vi "LEBITplc.TestIonSourceMonitor.vi"(0 "i ref in":refnum<vi>, 1 "data":i8[](array[numeric]), 2 "i attribute in":T1, 3 "index":i32, 4 "NickNames":string, 5 "error in":errorcluster, 7 "no link":bool) -> (14 "i ref out":refnum<vi>, 15 "Data":dbl[](array[numeric]), 16 "i attribute out":T1, 17 "Indexs":i32[](array[numeric]), 19 "error out":errorcluster)   [LabVIEW 2014, in "LEBITplc.lvlib"]
uses:
  LEBITplc.lvlib
  LEBITplc.i attribute.ctl
panel:
  out "No Link":bool
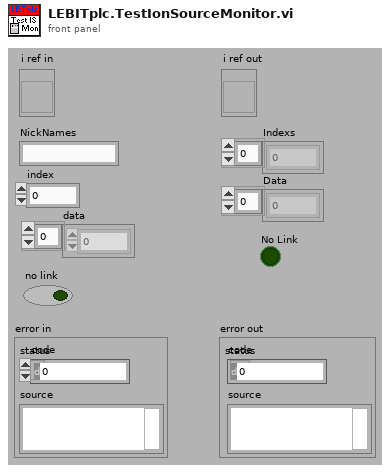
[diagram p1: front panel]
types:
  T1 = typedef "LEBITplc.lvlib/LEBITplc.i attribute.ctl" = cluster{"LLFLocation":string, "SetFileLocation":string, "nickNames":string[], "setValuePLCServiceID":i32[], "GUIServiceID":i32[], "monValuePLC":string[], "SetValueServiceID":i32[], "MonValueServiceID":i32[], "SetValue":dbl[][], "SetValueMin":dbl[], "SetValueMax":dbl[], "SetValueInfoServiceID":i32[], "GUINames":string[], "ListOfBases":string[], "Scale":dbl[], "Offset":dbl[], "setValuePLC":string[], "BaseName":string[], "ScaleServiceID":i32[], "OffsetServiceID":i32[], "AllPLCValues":string[], "CondSpecialArray":string[][], "CondSpecialIndex":i32[], "CondSpecialMonValue":dbl[], "RecentlyChanged":i32[], "SetFileLocationID":i32, "Dependent-Monitors":string[][], "LastLoadedFiles":string[], "IonGuideCalibLocation":string, "Monitor Dependent":string[], "Special":string[], "PLC?":bool[], "Start Date":string, "ListOfBasesServiceID":i32, "SETRA VISA resource":refnum<visa-resource-name>}
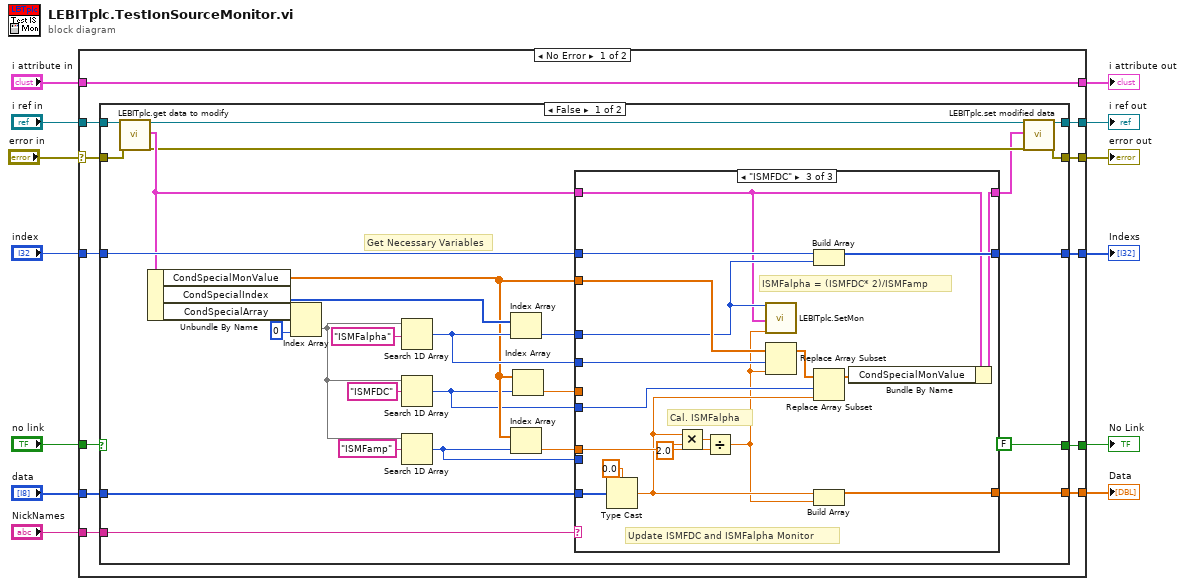
[diagram p0: block diagram]
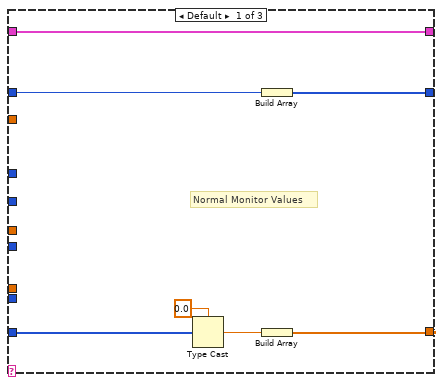
[diagram p2: hidden frame]
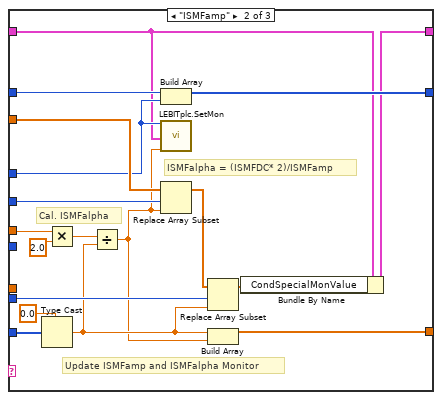
[diagram p3: hidden frame]
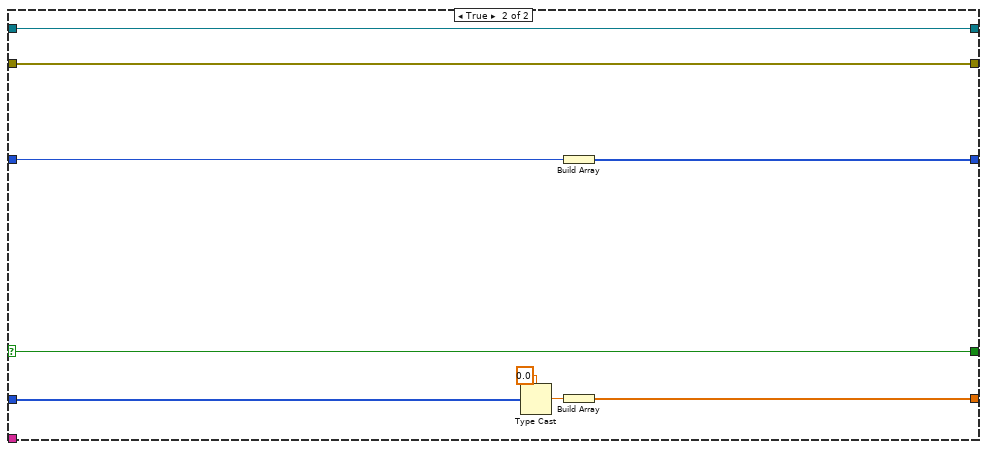
[diagram p4: hidden frame]
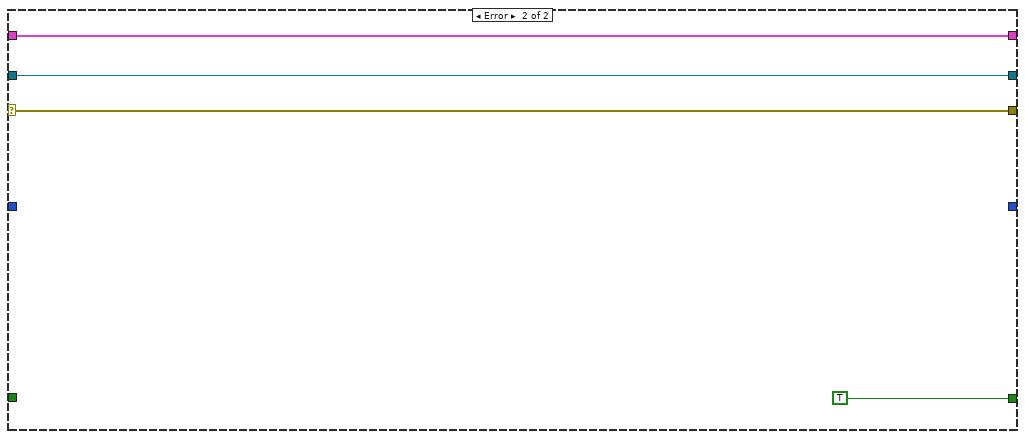
[diagram p5: hidden frame]
diagram:
  n1 = case shown="No Error" "error in" {
    selector: "error in" -> [w19 w109]
    tunnel: "NickNames" -> [w25 _]
    tunnel: [w20 w109] -> w12
    tunnel: "data" -> [w24 _]
    tunnel: "i attribute in" -> [w16 w107]
    tunnel: "i ref in" -> [w21 w108]
    tunnel: [w15 w108] -> w7
    tunnel: "index" -> [w23 _]
    tunnel: [w16 w107] -> w5
    tunnel: [w22 _] -> w4
    tunnel: "no link" -> [w18 _]
    tunnel: [w17 TRUE] -> w2
    tunnel: [w14 _] -> w1
    frame No Error {
      n2 = case shown="False" w18 {
        selector: w18 -> [_ w103]
        tunnel: w25 -> [w50 _]
        tunnel: w24 -> [w49 w99]
        tunnel: w23 -> [w42 w102]
        tunnel: [w41 w101] -> w22
        tunnel: w21 -> [w34 w105]
        tunnel: [w28 w105] -> w15
        tunnel: [w29 w104] -> w20
        tunnel: w19 -> [w32 w104]
        tunnel: [FALSE w103] -> w17
        tunnel: [w26 w97] -> w14
        frame False {
          # "Get Necessary Variables"
          n3 = call "LEBITplc.get data to modify.vi"("i ref in"=w34, "error in (no error)"=w32) -> ("i ref out"=w31:refnum<vi>, "i attribute"=w33:T1, "error out"=w30:errorcluster)  [unwired: 14 in, 1 out]
          n4 = Unbundle By Name(w33) -> ("CondSpecialMonValue"=w38:dbl[], "CondSpecialIndex"=w45:i32[], "CondSpecialArray"=w53:string[][])
          n5 = Index Array(array=w53, index (col)=0 ("index (row)")) -> (element=w44:string[])  [unwired: 1 in]
          n6 = Search 1D Array(1D array=w44, element="ISMFalpha") -> (index of element=w39:i32)  [unwired: 1 in]
          n7 = Search 1D Array(1D array=w44, element="ISMFDC") -> (index of element=w36:i32)  [unwired: 1 in]
          n8 = Search 1D Array(1D array=w44, element="ISMFamp") -> (index of element=w37:i32)  [unwired: 1 in]
          n9 = Index Array(array=w45, index=w39) -> (element=w43:i32)
          n10 = Index Array(array=w38, index=w37) -> (element=w46:dbl)
          n11 = Index Array(array=w38, index=w36) -> (element=w47:dbl)
          n12 = case shown="\"ISMFDC\"" w50 {
            tunnel: w49 -> [w57 w76 w94]
            tunnel: w47 -> [_ w68 _]
            tunnel: w46 -> [_ _ w85]
            tunnel: w43 -> [_ w62 w81]
            tunnel: w42 -> [w59 w77 w95]
            tunnel: [w60 w75 w93] -> w41
            tunnel: w33 -> [w54 w61 w80]
            tunnel: [w54 w70 w89] -> w27
            tunnel: w39 -> [_ w74 w92]
            tunnel: w38 -> [_ w69 w88]
            tunnel: w37 -> [_ w73 _]
            tunnel: w36 -> [_ _ w86]
            tunnel: [w55 w64 w82] -> w26
            frame Default {
              # "Normal Monitor Values"
              n13 = Type Cast(type=0.0 ("y"), x=w57) -> (*(type *) &x=w56:dbl)
              n14 = Build Array(w59) -> (w60:i32[])
              n15 = Build Array(w56) -> (w55:dbl[])
            }
            frame "ISMFamp" {
              # "ISMFalpha = (ISMFDC* 2)/ISMFamp"
              # "Cal. ISMFalpha"
              # "Update ISMFamp and ISMFalpha Monitor"
              n16 = Type Cast(type=0.0 ("y"), x=w76) -> (*(type *) &x=w65:dbl)
              n17 = Multiply(x=w68, y=2.0) -> (x*y=w66:dbl)
              n18 = Divide(x=w66, y=w65) -> (x/y=w63:dbl)
              n19 = Build Array(w77, w62) -> (w75:i32[])
              n20 = call "LEBITplc.SetMon.vi"("index of element"=w62, "i attribute in"=w61, "Data"=w63) -> ()  [unwired: 17 in]
              n21 = Replace Array Subset(array=w69, new element=w63, index=w74) -> (w72:dbl[])
              n22 = Replace Array Subset(array=w72, new element=w65, index=w73) -> (w71:dbl[])
              n23 = Build Array(w65, w63) -> (w64:dbl[])
              n24 = Bundle By Name(cluster=w61, "CondSpecialMonValue"=w71) -> (w70:T1)
            }
            frame "ISMFDC" {
              # "ISMFalpha = (ISMFDC* 2)/ISMFamp"
              # "Cal. ISMFalpha"
              # "Update ISMFDC and ISMFalpha Monitor"
              n25 = Type Cast(type=0.0 ("y"), x=w94) -> (*(type *) &x=w83:dbl)
              n26 = Multiply(x=w83, y=2.0) -> (x*y=w84:dbl)
              n27 = Divide(x=w84, y=w85) -> (x/y=w79:dbl)
              n28 = call "LEBITplc.SetMon.vi"("index of element"=w81, "i attribute in"=w80, "Data"=w79) -> ()  [unwired: 17 in]
              n29 = Replace Array Subset(array=w88, new element=w79, index=w92) -> (w91:dbl[])
              n30 = Build Array(w95, w81) -> (w93:i32[])
              n31 = Replace Array Subset(array=w91, new element=w83, index=w86) -> (w90:dbl[])
              n32 = Build Array(w83, w79) -> (w82:dbl[])
              n33 = Bundle By Name(cluster=w80, "CondSpecialMonValue"=w90) -> (w89:T1)
            }
          }
          n34 = call "LEBITplc.set modified data.vi"("i ref in"=w31, "i attribute"=w27, "error in (no error)"=w30) -> ("i ref out"=w28:refnum<vi>, "error out"=w29:errorcluster)  [unwired: 15 in]
        }
        frame True {
          n35 = Type Cast(type=0.0 ("y"), x=w99) -> (*(type *) &x=w98:dbl)
          n36 = Build Array(w102) -> (w101:i32[])
          n37 = Build Array(w98) -> (w97:dbl[])
        }
      }
    }
    frame Error {
    }
  }
  "error out" <- w12
  "i ref out" <- w7
  "i attribute out" <- w5
  "Indexs" <- w4
  "No Link" <- w2
  "Data" <- w1
